vi "VGap_GapDecrease.vi"(1 "error in (no error)":errorcluster, 2 "Step Decrease (um)":i32, 3 "Gap Decrease (um)":i32, 4 "System Index In":u32) -> (0 "error out":errorcluster)   [LabVIEW 2010]
panel:
  out "Current Step":i32
  out "Number of Step":dbl
  out "Position 3":dbl
  out "Position 2":dbl
  out "Position 1":dbl
  out "Initial Position 1 (um) 3":dbl
  out "Initial Position 1 (um) 2":dbl
  out "Initial Position 1 (um)":dbl
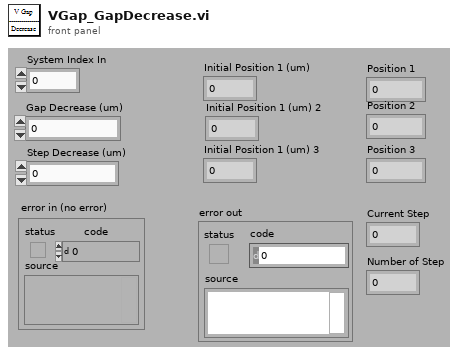
[diagram p1: front panel]
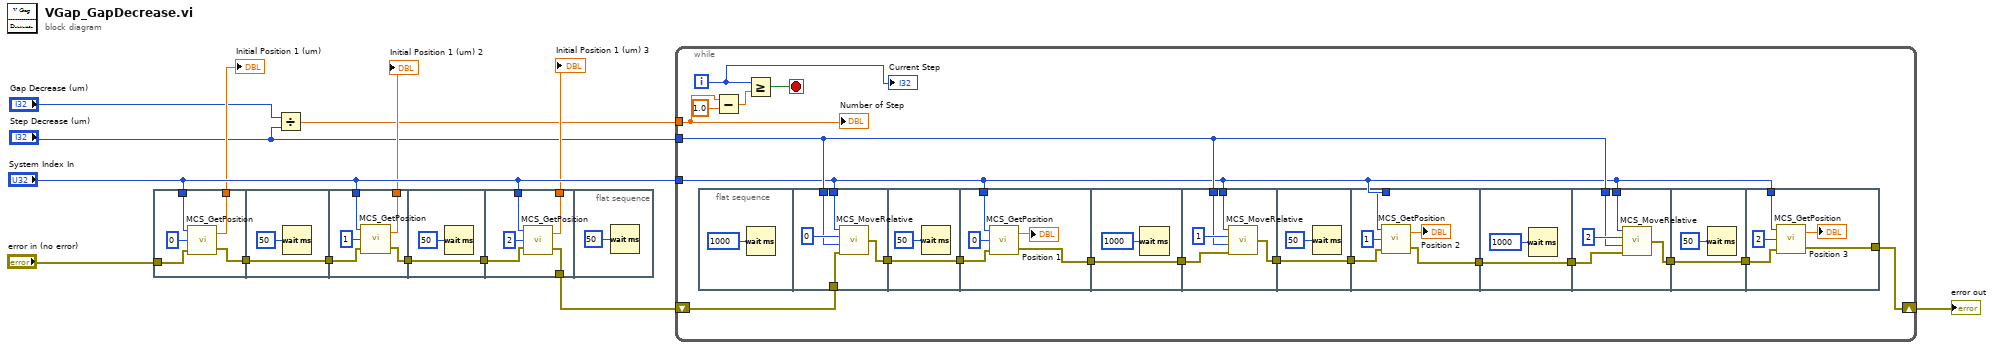
[diagram p0: block diagram]
diagram:
  n1 = flat-sequence {
    tunnel: "System Index In" -> [w18]
    tunnel: [w17] -> w13
    tunnel: [w16] -> w5
    tunnel: "error in (no error)" -> [w15]
    tunnel: [w20] -> w6
    tunnel: w5 -> [w20]
    tunnel: "System Index In" -> [w25]
    tunnel: [w24] -> w12
    tunnel: [w23] -> w7
    tunnel: w6 -> [w22]
    tunnel: [w27] -> w8
    tunnel: w7 -> [w27]
    tunnel: "System Index In" -> [w32]
    tunnel: [w31] -> w11
    tunnel: [w30] -> w9
    tunnel: w8 -> [w29]
    frame #0 {
      n2 = call "MCS_GetPosition.vi"("error in (no error)"=w15, "Channel Index In"=u32 0, "System Index In"=w18) -> ("error out"=w16:errorcluster, "Position (um)"=w17:dbl)
    }
    frame #1 {
      n3 = Wait (ms)(milliseconds to wait=u32 50) -> ()  [unwired: 1 out]
    }
    frame #2 {
      n4 = call "MCS_GetPosition.vi"("error in (no error)"=w22, "Channel Index In"=u32 1, "System Index In"=w25) -> ("error out"=w23:errorcluster, "Position (um)"=w24:dbl)
    }
    frame #3 {
      n5 = Wait (ms)(milliseconds to wait=u32 50) -> ()  [unwired: 1 out]
    }
    frame #4 {
      n6 = call "MCS_GetPosition.vi"("error in (no error)"=w29, "Channel Index In"=u32 2, "System Index In"=w32) -> ("error out"=w30:errorcluster, "Position (um)"=w31:dbl)
    }
    frame #5 {
      n7 = Wait (ms)(milliseconds to wait=u32 50) -> ()  [unwired: 1 out]
    }
  }
  n8 = Divide(x="Gap Decrease (um)", y="Step Decrease (um)") -> (x/y=w10:dbl)
  n9 = while {
    tunnel: "System Index In" -> [w51]
    tunnel: w10 -> [w36]
    tunnel: "Step Decrease (um)" -> [w52]
    shift-right: [w50] -> w3
    shift-left: w9 -> [w49]
    i -> [w35]
    stop <- w53 stop-if-true
    n10 = flat-sequence {
      tunnel: w51 -> [w59]
      tunnel: w52 -> [w57]
      tunnel: w49 -> [w56]
      tunnel: [w55] -> w47
      tunnel: [w60] -> w48
      tunnel: w47 -> [w60]
      tunnel: w51 -> [w65]
      tunnel: w48 -> [w63]
      tunnel: [w62] -> w45
      tunnel: [w67] -> w46
      tunnel: w45 -> [w67]
      tunnel: w51 -> [w72]
      tunnel: w52 -> [w71]
      tunnel: w46 -> [w70]
      tunnel: [w69] -> w43
      tunnel: [w74] -> w44
      tunnel: w43 -> [w74]
      tunnel: w51 -> [w79]
      tunnel: w44 -> [w77]
      tunnel: [w76] -> w41
      tunnel: [w81] -> w42
      tunnel: w41 -> [w81]
      tunnel: w51 -> [w86]
      tunnel: w52 -> [w85]
      tunnel: w42 -> [w84]
      tunnel: [w83] -> w39
      tunnel: [w88] -> w40
      tunnel: w39 -> [w88]
      tunnel: w51 -> [w93]
      tunnel: [w91] -> w50
      tunnel: w40 -> [w90]
      frame #0 {
        n11 = Wait (ms)(milliseconds to wait=u32 1000) -> ()  [unwired: 1 out]
      }
      frame #1 {
        n12 = call "MCS_MoveRelative.vi"("error in (no error)"=w56, "Moving Distance (um)"=w57, "Channel Index In"=u32 0, "System Index In"=w59) -> ("error out"=w55:errorcluster)
      }
      frame #2 {
        n13 = Wait (ms)(milliseconds to wait=u32 50) -> ()  [unwired: 1 out]
      }
      frame #3 {
        n14 = call "MCS_GetPosition.vi"("error in (no error)"=w63, "Channel Index In"=u32 0, "System Index In"=w65) -> ("error out"=w62:errorcluster, "Position (um)"=→"Position 1":dbl)
      }
      frame #4 {
        n15 = Wait (ms)(milliseconds to wait=u32 1000) -> ()  [unwired: 1 out]
      }
      frame #5 {
        n16 = call "MCS_MoveRelative.vi"("error in (no error)"=w70, "Moving Distance (um)"=w71, "Channel Index In"=u32 1, "System Index In"=w72) -> ("error out"=w69:errorcluster)
      }
      frame #6 {
        n17 = Wait (ms)(milliseconds to wait=u32 50) -> ()  [unwired: 1 out]
      }
      frame #7 {
        n18 = call "MCS_GetPosition.vi"("error in (no error)"=w77, "Channel Index In"=u32 1, "System Index In"=w79) -> ("error out"=w76:errorcluster, "Position (um)"=→"Position 2":dbl)
      }
      frame #8 {
        n19 = Wait (ms)(milliseconds to wait=u32 1000) -> ()  [unwired: 1 out]
      }
      frame #9 {
        n20 = call "MCS_MoveRelative.vi"("error in (no error)"=w84, "Moving Distance (um)"=w85, "Channel Index In"=u32 2, "System Index In"=w86) -> ("error out"=w83:errorcluster)
      }
      frame #10 {
        n21 = Wait (ms)(milliseconds to wait=u32 50) -> ()  [unwired: 1 out]
      }
      frame #11 {
        n22 = call "MCS_GetPosition.vi"("error in (no error)"=w90, "Channel Index In"=u32 2, "System Index In"=w93) -> ("error out"=w91:errorcluster, "Position (um)"=→"Position 3":dbl)
      }
    }
    n23 = Subtract(x=w36, y=1.0) -> (x-y=w38:dbl)
    n24 = Greater Or Equal?(x=w35, y=w38) -> (x >= y?=w53:bool)
    "Number of Step" <- w36
    "Current Step" <- w35
  }
  "error out" <- w3
  "Initial Position 1 (um)" <- w13
  "Initial Position 1 (um) 2" <- w12
  "Initial Position 1 (um) 3" <- w11
